vi "Parse Data JSON.vi"(8 "error in (no error)":errorcluster, 10 "Data JSON":string, 11 "Response in":refnum<class "Response.lvclass">) -> (0 "error out":errorcluster, 1 "Replaced?":bool, 2 "Typed Message":refnum<class "Response.lvclass">, 3 "Response out":refnum<class "Response.lvclass">)   [LabVIEW 2020, in "obs-websocket.lvlib" / "Response.lvclass"]
uses:
  Response.lvclass
  C:/dev/lv20CE/relink/lv-obs-websocket/obs-websocket/Server Message/Server Message.lvclass
  Response.lvclass/Response.ctl
  936e9ec3-f5c6-4689-99f4-a9412226f3da.vi
  <vilib>/JDP Science/JSONtext/Next JSON Value.vi
  <vilib>/JDP Science/JSONtext/String Subset.vi
  <vilib>/JDP Science/JSONtext/Parsing/Advance past next JSON Value (inlined COPY).vi
  <vilib>/JDP Science/JSONtext/Parsing/Advance past whitespace.vi
  <vilib>/JDP Science/JSONtext/Parsing/Advance past String.vi
  <vilib>/JDP Science/JSONtext/Parsing/Advance past Number.vi
  <vilib>/JDP Science/JSONtext/Parsing/Advance past Line Ending.vi
  RGetSourceScreenshot/RGetSourceScreenshot.lvclass
  C:/dev/lv20CE/relink/lv-obs-websocket/obs-websocket/Response/Response.lvclass
  RGetSceneList/RGetSceneList.lvclass
  RGetCurrentProgramScene/RGetCurrentProgramScene.lvclass
  RGetStreamStatus/RGetStreamStatus.lvclass
  RGetInputKindList/RGetInputKindList.lvclass
  RGetInputList/RGetInputList.lvclass
  RJSONDebug/RJSONDebug.lvclass
  RGetInputVolume/RGetInputVolume.lvclass
  REmptyResponse/REmptyResponse.lvclass
  RGetSceneItemID/RGetSceneItemID.lvclass
  RGetSceneItemEnabled/RGetSceneItemEnabled.lvclass
  RGetInputMute/RGetInputMute.lvclass
  <vilib>/JDP Science/JSONtext/JSON text to Variant.vi
  <vilib>/JDP Science/JSONtext/Parsing/Parse Full Path or Item Name.vi
  <vilib>/JDP Science/JSONtext/Parsing/Advance past Array.vi
  <vilib>/JDP Science/JSONtext/Parsing/Advance past Object.vi
  <vilib>/JDP Science/JSONtext/support/Error Cluster From Code.vi
  <vilib>/JDP Science/JSONtext/Offset/Find Item Locations by Path.vi
  <vilib>/JDP Science/JSONtext/LVClass Serializer/JSONtext LVClass Serializer.lvclass
  obs-websocket.lvlib
  <vilib>/JDP Science/JSONtext/JSONtext.lvlib
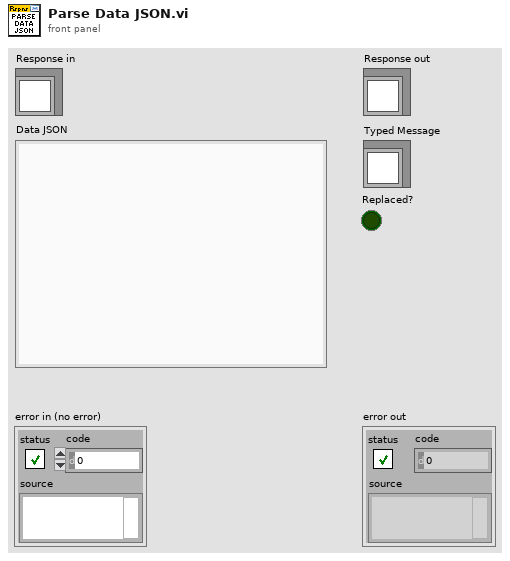
[diagram p1: front panel]
types:
  T1 = cluster{"requestType":string, "requestId":string, "requestStatus":cluster{"result":bool, "code":i32, "comment":string}}
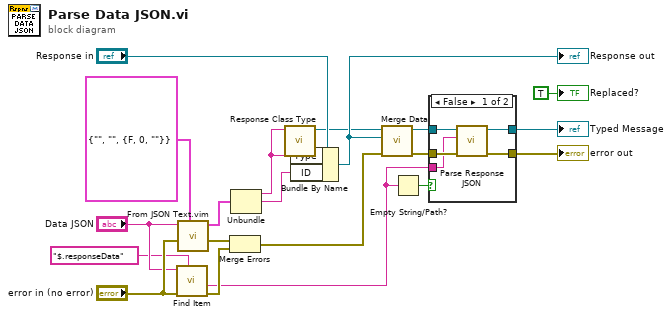
[diagram p0: block diagram]
diagram:
  n1 = call <vilib>:"Find Item.vi"("$Path or Item Name"="$.responseData", "error in (no error)"="error in (no error)", "JSON"="Data JSON") -> ("error out"=w7:errorcluster, "<JSON>"=w1:string)  [unwired: 5 in, 2 out]
  n2 = call "From JSON Text.vim"("Data Type and Default Value"=T1 {"requestType"="", "requestId"="", "requestStatus"={"result"=FALSE, "code"=0, "comment"=""}}, "error in (no error)"="error in (no error)", "JSON"="Data JSON") -> ("error out"=w8:errorcluster, "Data out"=w6:T1)  [unwired: 7 in]
  n3 = Merge Errors(w8, w7) -> (w3:errorcluster)
  n4 = Unbundle(w6) -> ("requestType"=w4:string, "requestId"=w5:string)  [unwired: 1 out]
  n5 = call "Response Class Type.vi"("Type"=w4) -> ("Class"=w12:refnum<class "Response.lvclass">)  [unwired: 10 in]
  n6 = Bundle By Name(cluster="Response in", "Type"=w4, "ID"=w5) -> (w15:refnum<class "Response.lvclass">)
  "Response out" <- w15
  n7 = call-dynamic "Merge Data.vi"("error in (no error)"=w3, "From"=w15, "Typed Response in"=w12) -> ("error out"=w17:errorcluster, "Typed Response out"=w18:refnum<class "Response.lvclass">)  [unwired: 7 in]
  n8 = Empty String/Path?(string/path=w1) -> (empty?=w2:bool)
  n9 = case shown="False" w2 {
    tunnel: w18 -> [w25 w27]
    tunnel: [w24 w27] -> w14
    tunnel: w17 -> [w23 w26]
    tunnel: [w22 w26] -> w16
    tunnel: w1 -> [w21 _]
    frame False {
      n10 = call-dynamic "Parse Response JSON.vi"("error in (no error)"=w23, "Response JSON"=w21, "Response in"=w25) -> ("error out"=w22:errorcluster, "Response out"=w24:refnum<class "Response.lvclass">)  [unwired: 7 in]
    }
    frame True {
    }
  }
  "error out" <- w16
  "Typed Message" <- w14
  "Replaced?" <- TRUE ("Replaced?")
